vi "Test_FormatValues_CommonTypes_ValuesOK.vi"(8 "error in (no error)":errorcluster, 11 "TestCase in":refnum<class "TestVariantExtensions.lvclass">) -> (0 "error out":errorcluster, 3 "TestCase out":refnum<class "TestVariantExtensions.lvclass">)   [LabVIEW 2020, in "TestVariantExtensions.lvclass"]
uses:
  TestVariantExtensions.lvclass
  Source/Scalar Data to String.vi
  <vilib>/Utility/Data Type/Get Type Information.vi
  <vilib>/Utility/Data Type/Get Numeric Information.vi
  <vilib>/Utility/Data Type/Get Refnum Information.vi
  TestVariantExtensions.lvclass/TestVariantExtensions.ctl
  Source/VariantExtensions.lvlib
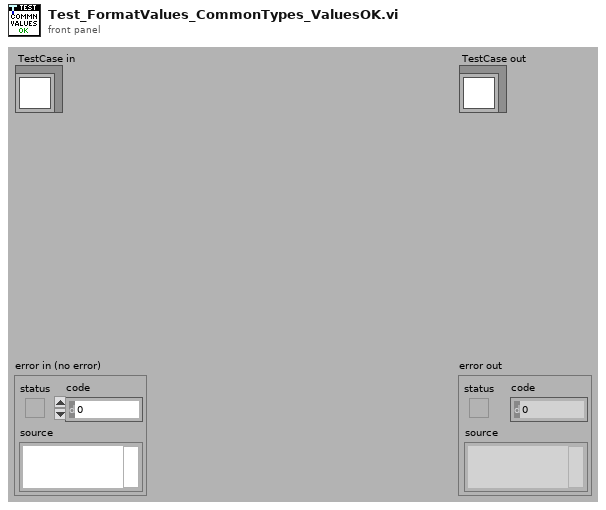
[diagram p1: front panel]
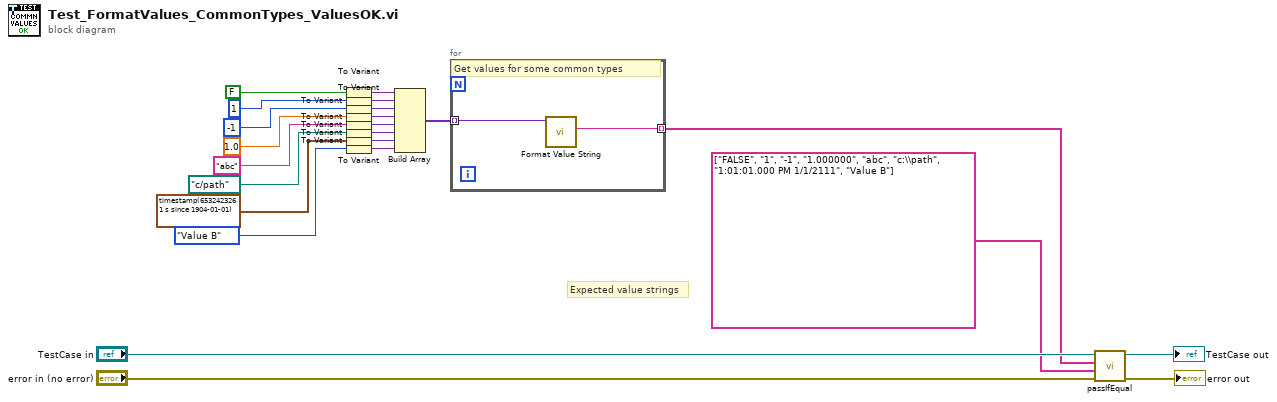
[diagram p0: block diagram]
diagram:
  # "Expected value strings"
  n1 = To Variant(anything=FALSE) -> (Variant=w4:variant)
  n2 = To Variant(anything=u32 1) -> (Variant=w19:variant)
  n3 = To Variant(anything=-1) -> (Variant=w18:variant)
  n4 = To Variant(anything=1.0) -> (Variant=w17:variant)
  n5 = To Variant(anything="abc") -> (Variant=w16:variant)
  n6 = To Variant(anything=path "c:/path") -> (Variant=w15:variant)
  n7 = To Variant(anything=timestamp(6532423261 s since 1904-01-01)) -> (Variant=w14:variant)
  n8 = To Variant(anything=enum16{"Value A", "Value B", "Value C"}."Value B") -> (Variant=w2:variant)
  n9 = Build Array(w4, w19, w18, w17, w16, w15, w14, w2) -> (w7:variant[])
  n10 = for {
    tunnel: [w25] -> w6 mode=indexing
    tunnel: w7 -> [w24] mode=indexing
    # "Get values for some common types"
    n11 = call "Format Value String.vi"("Data"=w24) -> ("Value as String"=w25:string)  [unwired: 9 in, 1 out]
  }
  n12 = call-dynamic "passIfEqual.vi"("error in (no error)"="error in (no error)", "y"=string[] ["FALSE", "1", "-1", "1.000000", "abc", "c:\\path", "1:01:01.000 PM 1/1/2111", "Value B"] ("Array"), "x"=w6, "TestCase in"="TestCase in") -> ("error out"=→"error out":errorcluster, "TestCase out"=→"TestCase out":refnum<class "TestVariantExtensions.lvclass">)  [unwired: 6 in]
